vi "HovaCal Stufen aufteilen.vi"(8 "error in (no error)":errorcluster caption="Fehler (Eingang, kein Fehler)") -> (0 "error out":errorcluster caption="Fehler (Ausgang)", 1 "Stufen":dbl[](array[numeric]), 2 "Gasnummer:":u8, 3 "Stufen":u16[](array[numeric]))   [LabVIEW 2020, in "Linearisierung v2.lvlib" / "Gasteiler.lvlib" / "HovaCal.lvlib"]
uses:
  HovaCal.lvlib
  Aktionen FGV Gasteiler Daten.ctl
  Aktion Lin Daten aufarbeiten.ctl
  Gasteiler.lvlib
  Linearisierung v2.lvlib
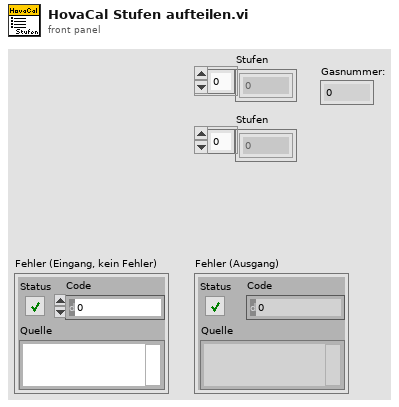
[diagram p1: front panel]
types:
  T1 = typedef "Linearisierung v2.lvlib/Aktion Lin Daten aufarbeiten.ctl" = enum16{"lesen", "Protkolldaten", "speichern", "laden", "EPA auswerten", "Tabelle schreiben", "Lin auswerten", "Tab init", "Stufentabelle", "EPA aktiviert", "Nachbehandlung laden", "Tabelle löschen", "Istwerte löschen", "Zeile löschen", "Zeile einfügen", "LIN aktiviert", "LIN/EPA aktiv laden", "EGAK Tab", "LIN übernehmen", "Tab init ohne Stufen"}
  T2 = typedef "Linearisierung v2.lvlib/Gasteiler.lvlib/Aktionen FGV Gasteiler Daten.ctl" = enum16{"lesen", "Gasteiler Daten", "Seriellen Param.", "MB-Endwert", "laden", "speichern", "Anforderung", "TCP", "Aufzeichnung Start"}
  T3 = typedef "Linearisierung v2.lvlib/Lin-Polynom Daten.ctl" = cluster{"Messgerät":string, "Kalibrator (Gasteiler)":string, "Bearbeiter/in":string, "Komponente":string, "Zeitstempel":timestamp, "F_max gefordert (%)":sgl, "F_max in %":sgl, "F_max in ppm":sgl, "Vorschlag Ordnung":i32, "Polynom OK":bool, "Polynomkoeff.":dbl[], "Prüfgas Konzentration":dbl, "Pfad EPA":string, "Pfad_LIN":string, "Gasnummer:":u8, "Komponentenauswahl":T4, "Verdünnungsgas":T6, "Zeitdauer Stufe":T7, "Anzahl Stufen":T7, "F_max in % EPA":sgl, "F_max in ppm EPA":sgl, "F_max in % LIN":sgl, "F_max in ppm LIN":sgl, "Punkte umkehren":bool, "EPA Optionsfeld":T8, "Autolin Hovacal":T9, "Spanfactors":sgl[], "Kalibrierauswahl":T10, "Conditions:":T11, "Gasflaschen Nr.:":string, "Bottle Accuracy":dbl, "Konfig Gasflasche":T12, "Gasflasche":T13, "HovaCAL Flow AutoLin":T14, "MFC Output":T15, "Gas Ablaufdatum":timestamp, "Lin Modus":T16, "zusätzliche Zeitdauer Erster Punkt":sgl, "Offsets":sgl[]}
  T4 = typedef "Linearisierung v2.lvlib/KomponentenArray.ctl" = cluster{"Komponente:":T5, "Konzentration":dbl}[]
  T5 = typedef "Auswahlfeld.ctl" = u16
  T6 = typedef "Linearisierung v2.lvlib/Gasteiler.lvlib/Prüfgas in.ctl" = u16
  T7 = typedef "Zahlen-Eingabefeld.ctl" = sgl
  T8 = typedef "Linearisierung v2.lvlib/EPA Optionsfeld.ctl" = enum32{"Istwert", "Rohwert", "Linearisierter Wert"}
  T9 = typedef "Linearisierung v2.lvlib/Gasteiler.lvlib/HovaCal.lvlib/AutoLin Hovacal.ctl" = enum32{"Keine Auswahl", "Optionsauswahl 1", "Optionsauswahl 2"}
  T10 = typedef "Linearisierung v2.lvlib/Kalibrieroption.ctl" = u16
  T11 = typedef "Linearisierung v2.lvlib/Linearity verification 1065-307.lvlib/Condition.ctl" = u16
  T12 = typedef "System Einstellungen V2.lvlib/Konfig Gasflasche.ctl" = bool
  T13 = typedef "System Einstellungen V2.lvlib/Gasflasche Auswahl.ctl" = u16
  T14 = typedef "Linearisierung v2.lvlib/Gasteiler.lvlib/HovaCAL_Interface.lvlib/Controls.lvlib/Flow Einstellung.ctl" = cluster{"HovaCAL Flow Input Cluster":dbl}
  T15 = typedef "Linearisierung v2.lvlib/Gasteiler.lvlib/HovaCAL_Interface.lvlib/Controls.lvlib/Pump state.ctl" = cluster{"Run":bool}
  T16 = typedef "CalGas Aufschaltung.lvlib/Lin Modus.ctl" = u16
  T17 = typedef "Linearisierung v2.lvlib/Gasteiler.lvlib/Gasteiler Daten.ctl" = cluster{"Gasteiler":T18, "Gasteiler Stufen":T19, "Gasteiler Type":T20, "Konfig Gasteiler":T21, "Gasteiler Span Eingänge":u16}
  T18 = typedef "String - Eingabefeld.ctl" = string
  T19 = typedef "Linearisierung v2.lvlib/Gasteiler.lvlib/Gasteiler Stufen.ctl" = u16
  T20 = typedef "Linearisierung v2.lvlib/GasteilerType.ctl" = u16
  T21 = typedef "System Einstellungen V2.lvlib/Gasteiler Auswahl.ctl" = u16
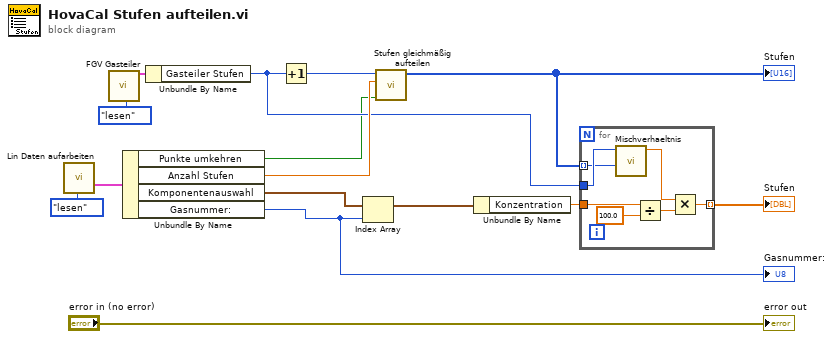
[diagram p0: block diagram]
diagram:
  n1 = call "Lin Daten aufarbeiten.vi"("Aktionen"=Aktion_Lin_Daten_aufarbeiten."lesen") -> ("Lin-Polynom"=w12:T3)  [unwired: 16 in, 10 out]
  n2 = call "FGV Gasteiler.vi"("Aktionen"=Aktionen_FGV_Gasteiler_Daten."lesen") -> ("Gasteiler Daten"=w14:T17)  [unwired: 11 in, 7 out]
  n3 = Unbundle By Name(w12) -> ("Punkte umkehren"=w2:bool, "Anzahl Stufen"=w7:T7, "Komponentenauswahl"=w9:T4, "Gasnummer:"=w3:u8)
  "Gasnummer:" <- w3
  n4 = Unbundle By Name(w14) -> ("Gasteiler Stufen"=w6:T19)
  n5 = Increment(x=w6) -> (x+1=w10:T19)
  n6 = Index Array(array=w9, index=w3) -> (element=w4:cluster{"Komponente:":T5, "Konzentration":dbl})
  n7 = call "Stufen gleichmäßig aufteilen.vi"("Punkte umkehren"=w2, "Stufen"=w7, "Anzahl"=w10) -> ("Stufen"=w11:u16[])  [unwired: 8 in]
  "Stufen" <- w11
  n8 = Unbundle By Name(w4) -> ("Konzentration"=w5:dbl)
  n9 = for {
    tunnel: w11 -> [w21] mode=indexing
    tunnel: w6 -> [w22]
    tunnel: w5 -> [w20]
    tunnel: [w16] -> w8 mode=indexing
    n10 = call "Mischverhaeltnis.vi"("Konzentration"=w21, "Sollwert"=w22) -> ("%"=w17:dbl)  [unwired: 8 in, 1 out]
    n11 = Divide(x=w20, y=sgl 100.0) -> (x/y=w18:dbl)
    n12 = Multiply(x=w17, y=w18) -> (x*y=w16:dbl)
  }
  "Stufen" <- w8
  "error out" <- "error in (no error)"
